vi "Temp Folder.vi"(3 "Relative Path (\"\")":string) -> (1 "Temp Folder":path)   [LabVIEW 2011]
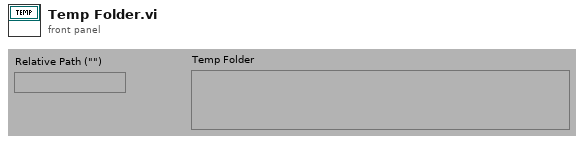
[diagram p1: front panel]
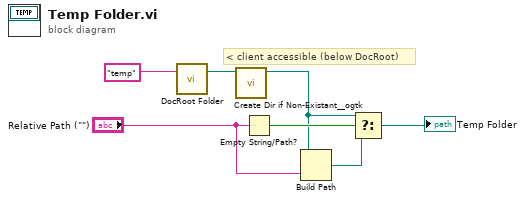
[diagram p0: block diagram]
diagram:
  # "< client accessible (below DocRoot)"
  n1 = call "DocRoot Folder.vi"("Relative Path (\"\" - Folder)"="temp" ("name or relative path")) -> ("DocumentRoot Folder"=w2:path)  [unwired: 2 in]
  n2 = call "Create Dir if Non-Existant__ogtk.vi"("Directory Path"=w2) -> ("dup Directory Path"=w3:path)  [unwired: 2 in, 8 out]
  n3 = Empty String/Path?(string/path="Relative Path (\"\")") -> (empty?=w6:bool)
  n4 = Build Path(base path=w3, name or relative path="Relative Path (\"\")") -> (appended path=w4:path)
  n5 = Select(t=w3, s=w6, f=w4) -> (s? t:f=→"Temp Folder":path)
